vi "AutoParser2.vi"() -> ()   [LabVIEW 2019]
panel:
  out "Parsed parameters":string[](array[string])
  in  "Parameters":string
  # "Parsed Parameters"
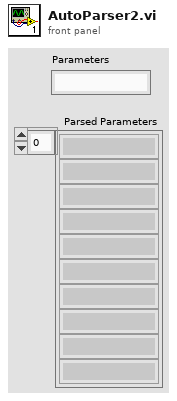
[diagram p1: front panel]
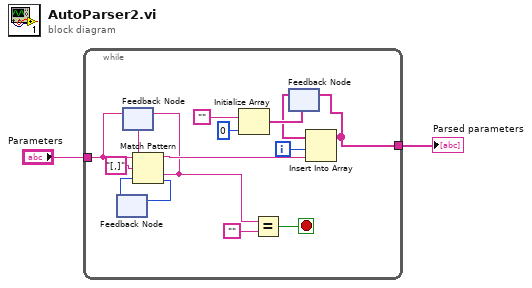
[diagram p0: block diagram]
diagram:
  n1 = while {
    tunnel: [w5] -> _
    tunnel: [w7] -> w2
    tunnel: "Parameters" -> [w4]
    i -> [w14]
    stop <- w16 stop-if-true
    n2 = feedback #1() -> (w12:i32)  [unwired: 1 in]
    n3 = feedback #2(w4) -> (w5:string)
    n4 = Match Pattern(string=w5, regular expression="[,]", offset (0)=w12) -> (before substring=w6:string, after substring=w3:string, offset past match=w13:i32)  [unwired: 1 out]
    n5 = feedback-in #1(w13) -> ()
    n6 = feedback-in #2(w3) -> ()
    n7 = Initialize Array("", 0 ("dimension size")) -> (w11:string[])
    n8 = Equal?(x=w3, y="") -> (x = y?=w16:bool)
    n9 = feedback #3(w11) -> (w8:string[])
    n10 = Insert Into Array(array=w8, index=w14, new element=w6) -> (w7:string[])
    n11 = feedback-in #3(w7) -> ()
  }
  "Parsed parameters" <- w2
